vi "Format Persistent Filename.vi"(9 "Datum Type":variant, 11 "Datum Name":string) -> (3 "Filename":string)   [LabVIEW 2020, in "MVA Framework.lvlib" / "PersistToDiskTransport.lvclass"]
doc: "格式化保持文件名"
uses:
  PersistToDiskTransport.lvclass
  variant-extensions/Source/VariantExtensions.lvlib
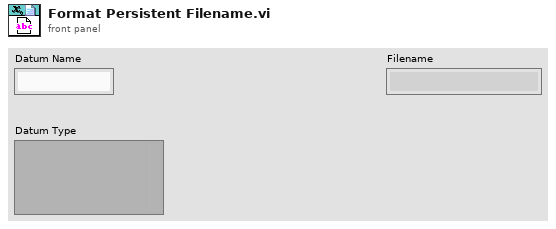
[diagram p1: front panel]
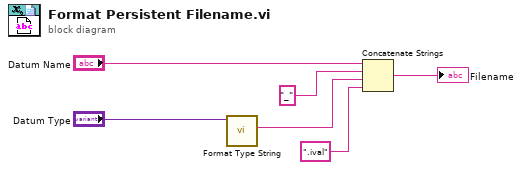
[diagram p0: block diagram]
diagram:
  n1 = call "Format Type String.vi"("Data Type"="Datum Type") -> ("Type Name"=w4:string)  [unwired: 9 in, 1 out]
  n2 = Concatenate Strings("Datum Name", "_" ("string"), w4, ".ival" ("string")) -> (→"Filename":string)
